vi "Wake_Up.vi"(8 "error in":errorcluster, 10 "timeout":dbl=10.0 format="%0.2f", 11 "DAQmx Task Name":refnum<k21>) -> (0 "error out":errorcluster)   [LabVIEW 2018]
panel:
  in  "Wake Up Time":dbl=3.0 caption="Time Target (s)"
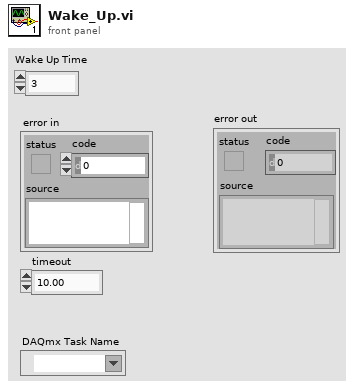
[diagram p1: front panel]
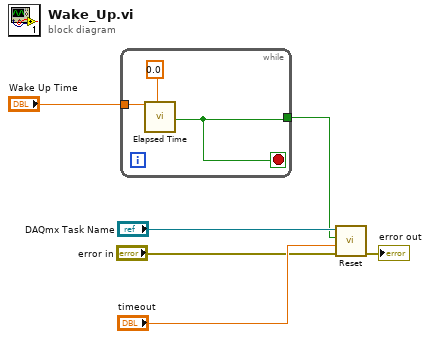
[diagram p0: block diagram]
diagram:
  n1 = while {
    tunnel: "Wake Up Time" -> [w8]
    tunnel: [w7] -> w1
    stop <- w7 stop-if-true
    n2 = call "Elapsed Time"("Time Target (s)"=w8, "Set Start Time (s)"=0.0) -> ("Time has Elapsed"=w7:bool)  [unwired: 10 in, 7 out]
  }
  n3 = call "Reset.vi"("error in"="error in", "timeout"="timeout", "Reset Logic Level"=w1, "DAQmx Task Name"="DAQmx Task Name") -> ("error out"=→"error out":errorcluster)  [unwired: 7 in]
